vi "Configure Waveform Modulation Function.vi"(6 "Waveform Rising Time (50)":dbl=50.0, 8 "error in (no error)":errorcluster, 9 "Modulating Signal Shape (0: Sinusoid)":i32(ring) items=["Sinusoid", "Square", "Ramp"], 10 "Waveform Generator Number (1 Waveform Generator 1)":i32(ring)=1 items=["Waveform Generator 1"=1], 11 "VISA resource name":refnum<visa-resource-name>) -> (0 "error out":errorcluster, 3 "VISA resource name out":refnum<visa-resource-name>)   [LabVIEW 2017, in "Agilent 2000 3000 X-Series.lvlib"]
doc: "Specifies the modulating waveform shape and the amount of time per cycle that it is rising."
uses:
  Agilent 2000 3000 X-Series.lvlib
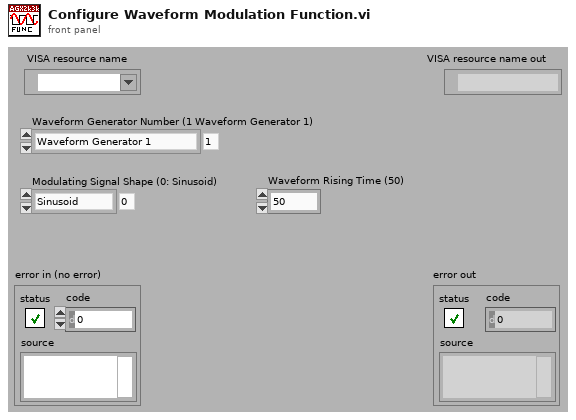
[diagram p1: front panel]
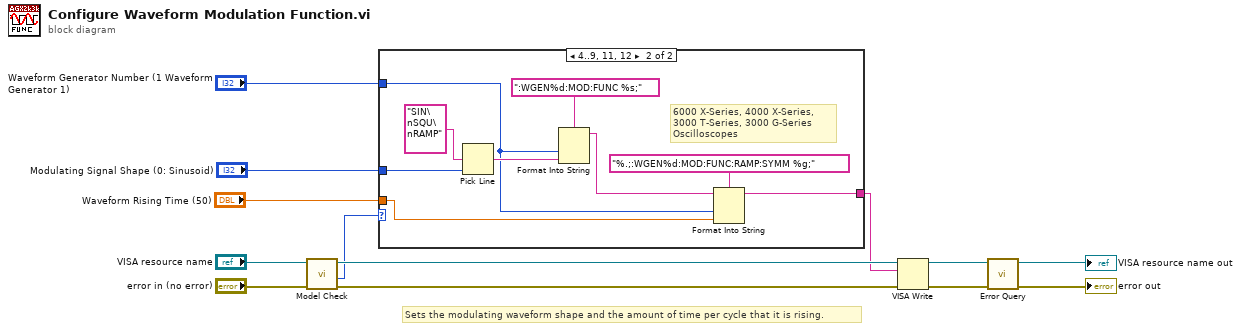
[diagram p0: block diagram]
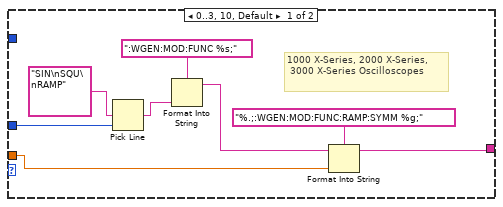
[diagram p2: hidden frame]
diagram:
  # "Sets the modulating waveform shape and the amount of time per cycle that it is rising."
  n1 = call "Model Check.vi"("error in (no error)"="error in (no error)", "VISA resource name"="VISA resource name") -> ("error out"=w10:errorcluster, "Model"=w5:i32, "VISA resource name out"=w11:refnum<visa-resource-name>)  [unwired: 7 out]
  n2 = case shown="4..9, 11, 12" w5 {
    tunnel: "Waveform Rising Time (50)" -> [w17 w26]
    tunnel: "Modulating Signal Shape (0: Sinusoid)" -> [w16 w25]
    tunnel: "Waveform Generator Number (1 Waveform Generator 1)" -> [_ w23]
    tunnel: [w18 w24] -> w1
    frame 0..3, 10, Default {
      # "1000 X-Series, 2000 X-Series,\n 3000 X-Series Oscilloscopes"
      n3 = Pick Line(multi-line string="SIN\nSQU\nRAMP", line index=w16) -> (output string=w15:string)  [unwired: 1 out]
      n4 = Format Into String(format string=":WGEN:MOD:FUNC %s;", w15) -> (resulting string=w14:string)  [unwired: 2 in, 1 out]
      n5 = Format Into String(format string="%.;:WGEN:MOD:FUNC:RAMP:SYMM %g;", initial string=w14, w17) -> (resulting string=w18:string)  [unwired: 1 in, 1 out]
    }
    frame 4..9, 11, 12 {
      # "6000 X-Series, 4000 X-Series, 3000 T-Series, 3000 G-Series Oscilloscopes"
      n6 = Pick Line(multi-line string="SIN\nSQU\nRAMP", line index=w25) -> (output string=w29:string)  [unwired: 1 out]
      n7 = Format Into String(format string=":WGEN%d:MOD:FUNC %s;", w23, w29) -> (resulting string=w28:string)  [unwired: 2 in, 1 out]
      n8 = Format Into String(format string="%.;:WGEN%d:MOD:FUNC:RAMP:SYMM %g;", initial string=w28, w23, w26) -> (resulting string=w24:string)  [unwired: 1 in, 1 out]
    }
  }
  n9 = VISA Write(VISA resource name=w11, write buffer=w1, error in (no error)=w10) -> (VISA resource name out=w9:refnum<visa-resource-name>, error out=w8:errorcluster)  [unwired: 1 out]
  n10 = call "Error Query.vi"("error in (no error)"=w8, "VISA resource name"=w9) -> ("error out"=→"error out":errorcluster, "VISA resource name out"=→"VISA resource name out":refnum<visa-resource-name>)  [unwired: 6 in, 2 out]
